vi "Get Endstop Status.vi"(8 "error in (no error)":errorcluster, 11 "VISA resource name":refnum<visa-resource-name>) -> (0 "error out":errorcluster, 2 "End stop status":T1, 3 "VISA resource name out":refnum<visa-resource-name>)   [LabVIEW 2020, in "Marlin Instrument Driver.lvlib"]
doc: "Returns the current state of the configured X, Y, Z endstops. Takes into account any 'inverted endstop' settings, so one can confirm that the machine is interpreting the endstops correctly."
uses:
  <instrlib>/Marlin Instrument Driver/Marlin Instrument Driver.lvlib
  <instrlib>/Marlin Instrument Driver/Public/controls/end stop status.ctl
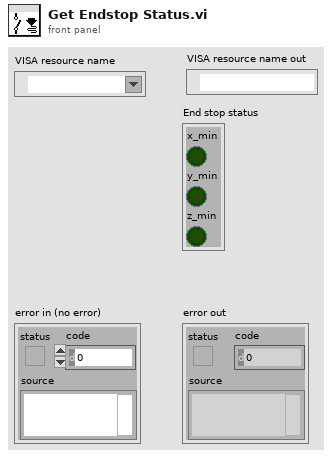
[diagram p1: front panel]
types:
  T1 = typedef "Marlin Instrument Driver.lvlib/end stop status.ctl" = cluster{"x_min":bool, "y_min":bool, "z_min":bool}
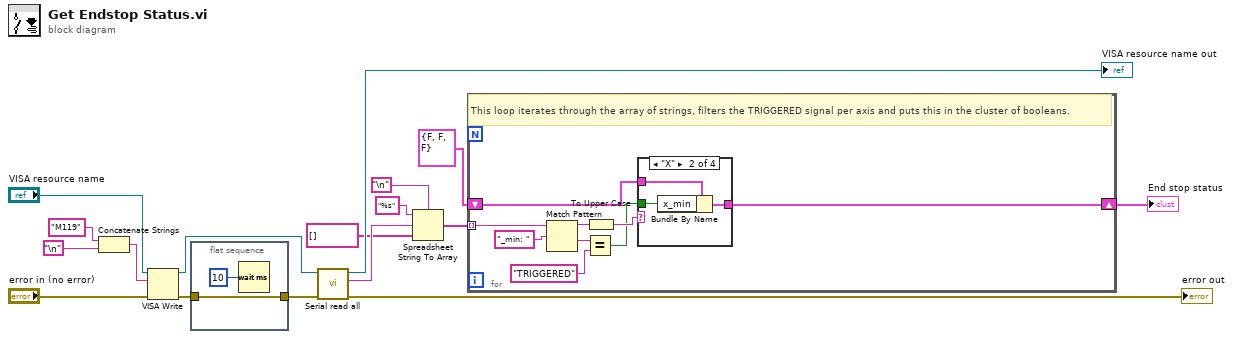
[diagram p0: block diagram]
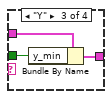
[diagram p3: hidden frame]
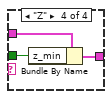
[diagram p4: hidden frame]
diagram:
  n1 = Concatenate Strings("M119" ("command"), "\n") -> (w14:string)
  n2 = VISA Write(VISA resource name="VISA resource name", write buffer=w14, error in (no error)="error in (no error)") -> (VISA resource name out=w13:refnum<visa-resource-name>, error out=w2:errorcluster)  [unwired: 1 out]
  n3 = flat-sequence {
    tunnel: w2 -> [w18]
    tunnel: [w18] -> w1
    frame #0 {
      n4 = Wait (ms)(milliseconds to wait=u32 10) -> ()  [unwired: 1 out]
    }
  }
  n5 = call <instrlib>:"Serial read all.vi"("error in (no error)"=w1, "VISA Refnum in"=w13) -> ("error out"=→"error out":errorcluster, "read buffer"=w9:string, "VISA Refnum out"=→"VISA resource name out":refnum<visa-resource-name>)  [unwired: 6 in, 1 out]
  n6 = Spreadsheet String To Array(delimiter (Tab)="\n", format string="%s", spreadsheet string=w9, array type (2D Dbl)=string[] []) -> (array=w7:string[])
  n7 = for {
    tunnel: w7 -> [w28] mode=indexing
    shift-right: [w21] -> w5
    shift-left: T1 {"x_min"=FALSE, "y_min"=FALSE, "z_min"=FALSE} ("End stop status") -> [w22]
    # "This loop iterates through the array of strings, filters the TRIGGERED signal per axis and puts this in the cluster of booleans."
    n8 = Match Pattern(string=w28, regular expression="_min: ") -> (before substring=w26:string, after substring=w24:string)  [unwired: 1 in, 2 out]
    n9 = Equal?(x=w24, y="TRIGGERED") -> (x = y?=w20:bool)
    n10 = To Upper Case(1:w26) -> (0:w25:string)
    n11 = case shown="\"X\"" w25 {
      tunnel: w22 -> [w29 w32 w35 w38]
      tunnel: [w29 w31 w34 w37] -> w21
      tunnel: w20 -> [_ w30 w33 w36]
      frame Default {
      }
      frame "X" {
        n12 = Bundle By Name(cluster=w32, "x_min"=w30) -> (w31:T1)
      }
      frame "Y" {
        n13 = Bundle By Name(cluster=w35, "y_min"=w33) -> (w34:T1)
      }
      frame "Z" {
        n14 = Bundle By Name(cluster=w38, "z_min"=w36) -> (w37:T1)
      }
    }
  }
  "End stop status" <- w5
